vi "Breath.vi"() -> ()   [LabVIEW 2022 SP3]
uses:
  <vilib>/Analysis/NI_AALPro.lvlib
  <vilib>/Analysis/2dsp.llb/1D Cross Correlation (DBL).vi
  <vilib>/Analysis/NI_AALBase.lvlib
  <vilib>/Analysis/baseanly.llb/Mean (DBL).vi
panel:
  in  "ExitSendCmd 2":bool
  in  "Folder to place data":path
  in  "Extra Pts for Corr":i32=250
  out "ROI Coords":T1
  in  "ExitSendCmd":bool
  out "Focus RF Pt":dbl
  out "Correlations for window":dbl[][](graph)
  out "Total RF shift for groups of 5":dbl[](graph)
  in  "ROC (mm)":i32=12
  out "Ref Image":dbl[][](graph)
  in  "Folder of data":path
  in  "pattern":string="*.eye"
  # "Only use with single sets of 25 in a folder for now."
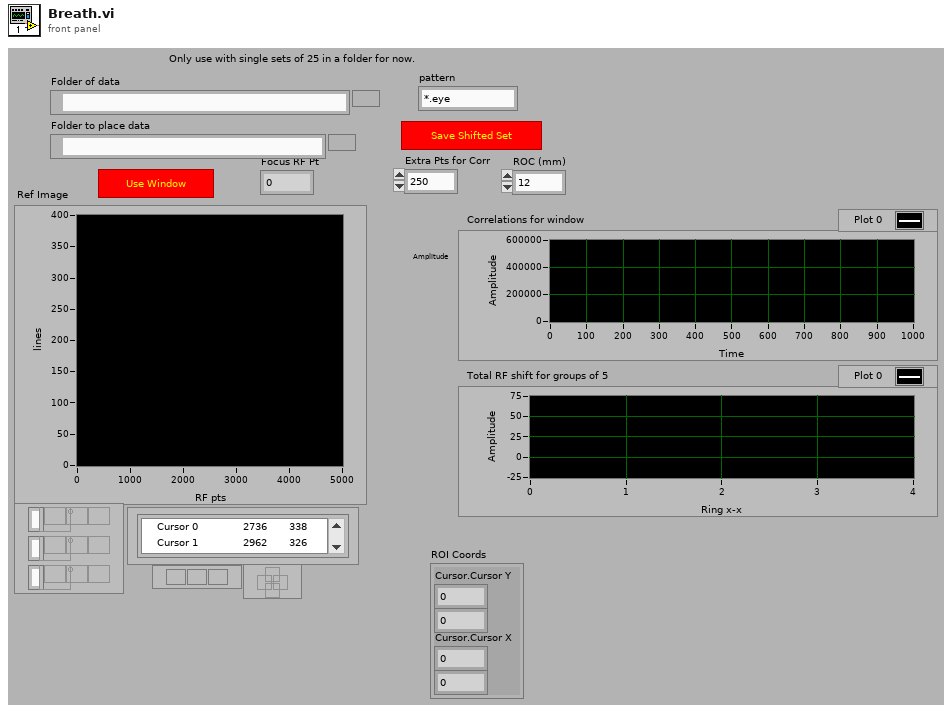
[diagram p1: front panel]
types:
  T1 = cluster{"Cursor.Cursor Y":dbl, dbl, "Cursor.Cursor X":dbl, dbl}
  T2 = cluster{"# rf points per line":u16, "# lines per scan":u16, "sample rate MHz":u16, "# A/D bits":u16, "# bytes per A/D":u16, "TGC Flag":u16, "A/D Type":string}
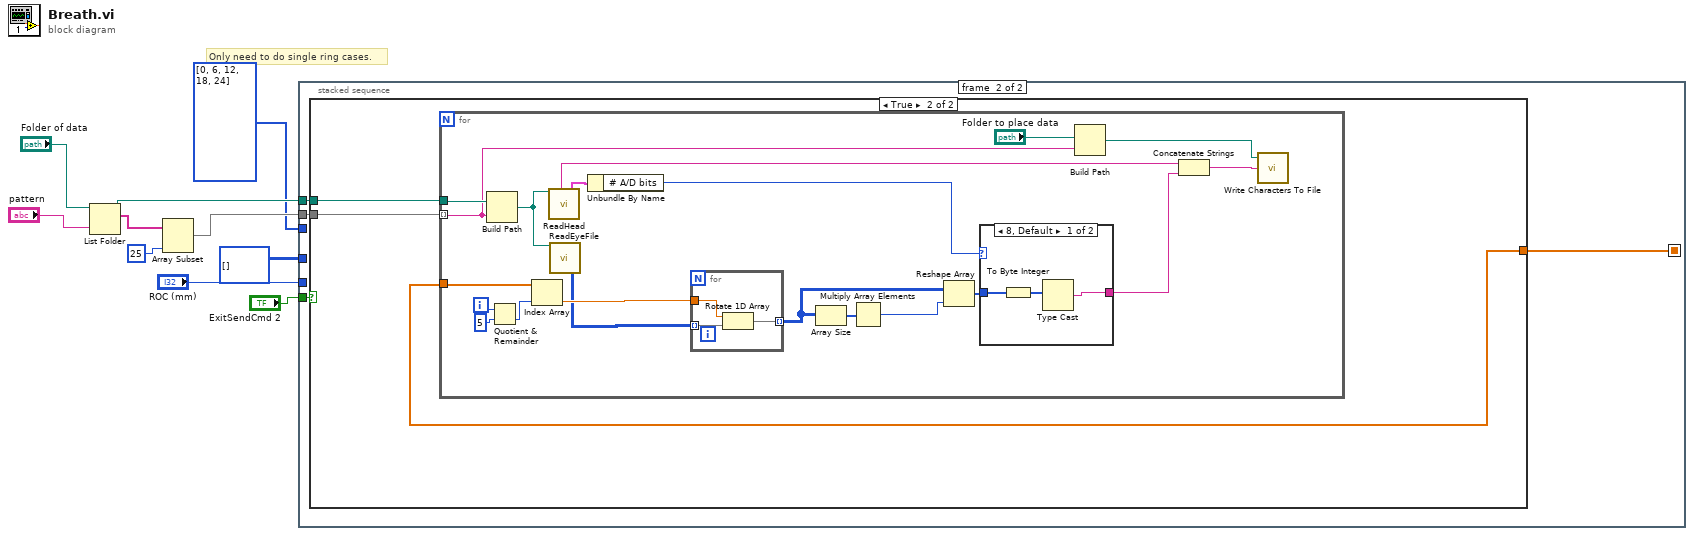
[diagram p0: block diagram]
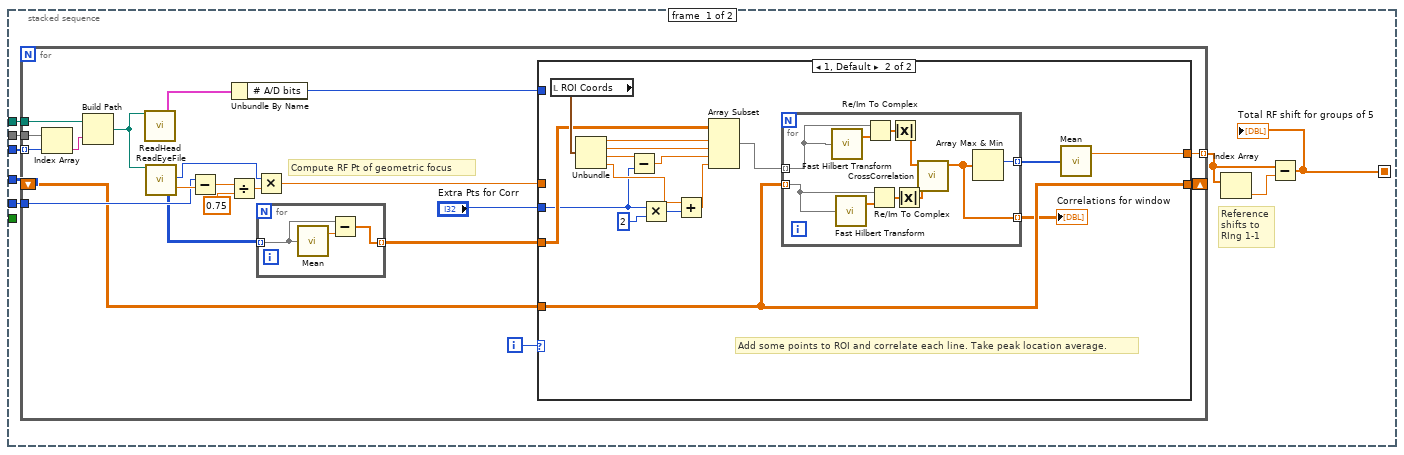
[diagram p2: hidden frame]
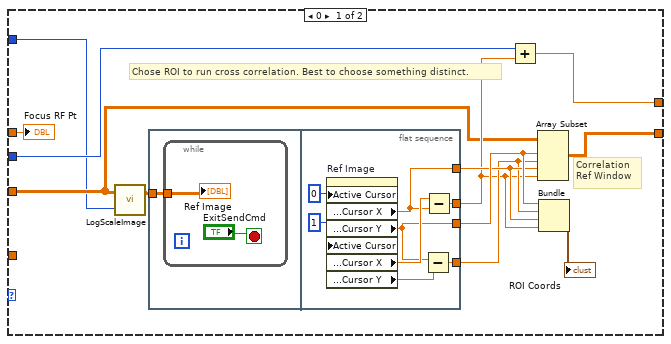
[diagram p3: hidden frame]
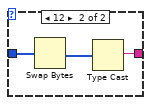
[diagram p5: hidden frame]
diagram:
  # "Only need to do single ring cases."
  n1 = List Folder(path="Folder of data", pattern="pattern") -> (path out=w8:path, filenames=w6:string[])  [unwired: 1 in, 3 out]
  n2 = Array Subset(array=w6, length=25) -> (w3:string[])  [unwired: 1 in]
  n3 = stacked-sequence {
    seq-local: [w11 _] -> [_ w93]
    tunnel: w8 -> [w18 w94]
    tunnel: "ROC (mm)" -> [w17 _]
    tunnel: i16[][] [] -> [w16 _]
    tunnel: w3 -> [w15 w95]
    tunnel: i32[] [0, 6, 12, 18, 24] -> [w14 _]
    tunnel: "ExitSendCmd 2" -> [_ w92]
    frame #0 {
      # "Reference shifts to RIng 1-1"
      n4 = for {
        tunnel: w15 -> [w22]
        tunnel: w18 -> [w39]
        tunnel: w17 -> [w35]
        shift-right: [w29] -> _
        shift-left: w16 -> [w28]
        tunnel: [w27] -> w12 mode=indexing
        tunnel: w14 -> [w20] mode=indexing
        i -> [w30]
        # "Compute RF Pt of geometric focus"
        n5 = Index Array(array=w22, index=w20) -> (element=w21:string)
        n6 = Build Path(base path=w39, name or relative path=w21) -> (appended path=w37:path)
        n7 = call "ReadHead.vi"("new file path"=w37) -> ("A/D info"=w38:T2)  [unwired: 18 out]
        n8 = call "ReadEyeFile.vi"("new file path"=w37) -> ("2-D data array"=w19:i16[][], "sample rate MHz"=w31:u16, "delay"=w36:sgl)  [unwired: 1 in, 15 out]
        n9 = Subtract(x=w35, y=w36) -> (x-y=w34:sgl)
        n10 = Divide(x=w34, y=0.75) -> (x/y=w32:dbl)
        n11 = Unbundle By Name(w38) -> ("# A/D bits"=w24:u16)
        n12 = Multiply(x=w31, y=w32) -> (x*y=w26:dbl)
        n13 = for {
          tunnel: [w41] -> w23 mode=indexing
          tunnel: w19 -> [w40] mode=indexing
          n14 = call-poly <vilib>:"Mean.vi"("X"=w40) -> ("mean"=w42:dbl)  [unwired: 1 out]
          n15 = Subtract(x=w40, y=w42) -> (x-y=w41:dbl[])
        }
        n16 = case shown="1, Default" w30 {
          tunnel: [w53 w81] -> w29
          tunnel: w28 -> [_ w81]
          tunnel: [w47 w80] -> w27
          tunnel: w26 -> [w54 _]
          tunnel: w23 -> [w45 w69]
          tunnel: "Extra Pts for Corr" -> [w49 w67]
          tunnel: w24 -> [w43 _]
          frame 0 {
            # "Correlation\nRef Window"
            # "Chose ROI to run cross correlation. Best to choose something distinct."
            n17 = call "LogScaleImage.vi"("A/D bits"=w43, "input array"=w45) -> ("log scale image"=w44:dbl[][])  [unwired: 1 out]
            n18 = flat-sequence {
              tunnel: w44 -> [w55]
              tunnel: [w61] -> w48
              tunnel: [w60] -> w52
              tunnel: [w59] -> w46
              tunnel: [w58] -> w51
              frame #0 {
                n19 = while {
                  tunnel: w55 -> [w56]
                  stop <- "ExitSendCmd" stop-if-true
                  "Ref Image" <- w56
                }
              }
              frame #1 {
                n20 = property on="Ref Image" class="IntGraph (strict)"("Active Cursor"=0, "Active Cursor"=1) -> ("Cursor.Cursor Position:Cursor X"=w58:dbl, "Cursor.Cursor Position:Cursor Y"=w60:dbl, "Cursor.Cursor Position:Cursor X"=w63:dbl, "Cursor.Cursor Position:Cursor Y"=w62:dbl)  [unwired: 2 in, 2 out]
                n21 = Subtract(x=w60, y=w62) -> (x-y=w61:dbl)
                n22 = Subtract(x=w63, y=w58) -> (x-y=w59:dbl)
              }
            }
            n23 = Add(x=w49, y=w46) -> (x+y=w47:dbl)
            n24 = Array Subset(array=w45, index (row)=w52, length (row)=w48, index (col)=w51, length (col)=w46) -> (w53:dbl[][])
            n25 = Bundle("Cursor.Cursor Y"=w52, w48, "Cursor.Cursor X"=w51, w46) -> (→"ROI Coords":T1)  [unwired: 1 out]
            "Focus RF Pt" <- w54
          }
          frame 1, Default {
            # "Add some points to ROI and correlate each line. Take peak location average."
            n26 = local read "ROI Coords"() -> (w78:T1)
            n27 = Unbundle(w78) -> ("Cursor.Cursor Y"=w77:dbl, w76:dbl, "Cursor.Cursor X"=w75:dbl, w71:dbl)
            n28 = Subtract(x=w75, y=w67) -> (x-y=w74:dbl)
            n29 = Multiply(x=w67, y=2) -> (x*y=w72:i32)
            n30 = Add(x=w71, y=w72) -> (x+y=w70:dbl)
            n31 = Array Subset(array=w69, index (row)=w77, length (row)=w76, index (col)=w74, length (col)=w70) -> (w68:dbl[][])
            n32 = for {
              tunnel: w68 -> [w84] mode=indexing
              tunnel: w81 -> [w85] mode=indexing
              tunnel: [w91] -> w79 mode=indexing
              tunnel: [w90] -> w66 mode=indexing
              n33 = call <vilib>:"Fast Hilbert Transform.vi"("X"=w84) -> ("Hilbert{X}"=w89:dbl[])  [unwired: 1 out]
              n34 = call <vilib>:"Fast Hilbert Transform.vi"("X"=w85) -> ("Hilbert{X}"=w87:dbl[])  [unwired: 1 out]
              n35 = Re/Im To Complex(1:w89, 2:w84) -> (0:w88:cdb[])
              n36 = Re/Im To Complex(1:w87, 2:w85) -> (0:w86:cdb[])
              n37 = Absolute Value(x=w88) -> (abs(x)=w83:dbl[])
              n38 = Absolute Value(x=w86) -> (abs(x)=w82:dbl[])
              n39 = call-poly <vilib>:"CrossCorrelation.vi"("Y"=w82, "X"=w83) -> ("Rxy"=w90:dbl[])  [unwired: 2 in, 7 out]
              n40 = Array Max & Min(array=w90) -> (max index (indices)=w91:i32)  [unwired: 3 out]
            }
            "Correlations for window" <- w66
            n41 = call-poly <vilib>:"Mean.vi"("X"=w79) -> ("mean"=w80:dbl)  [unwired: 1 out]
          }
        }
      }
      n42 = Index Array(array=w12) -> (element=w13:dbl)  [unwired: 1 in]
      n43 = Subtract(x=w12, y=w13) -> (x-y=w11:dbl[])
      "Total RF shift for groups of 5" <- w11
    }
    frame #1 {
      n44 = case shown="True" w92 {
        tunnel: w95 -> [_ w98]
        tunnel: w94 -> [_ w97]
        tunnel: w93 -> [_ w96]
        frame False {
        }
        frame True {
          n45 = for {
            tunnel: w98 -> [w102] mode=indexing
            tunnel: w97 -> [w117]
            tunnel: w96 -> [w108]
            i -> [w109]
            n46 = Build Path(base path=w117, name or relative path=w102) -> (appended path=w118:path)
            n47 = Quotient & Remainder(x=w109, y=5) -> (floor(x/y)=w107:i32)  [unwired: 1 out]
            n48 = Index Array(array=w108, index=w107) -> (element=w106:dbl)
            n49 = call "ReadHead.vi"("new file path"=w118) -> ("whole header"=w105:string, "A/D info"=w112:T2)  [unwired: 17 out]
            n50 = call "ReadEyeFile.vi"("new file path"=w118) -> ("2-D data array"=w99:i16[][])  [unwired: 1 in, 17 out]
            n51 = Unbundle By Name(w112) -> ("# A/D bits"=w111:u16)
            n52 = for {
              tunnel: w99 -> [w127] mode=indexing
              tunnel: [w126] -> w113 mode=indexing
              tunnel: w106 -> [w125]
              n53 = Rotate 1D Array(1:w127, 2:w125) -> (0:w126:i16[])
            }
            n54 = Array Size(array=w113) -> (size(s)=w115:i32[])
            n55 = Multiply Array Elements(1:w115) -> (0:w104:i32)
            n56 = Reshape Array(w113, w104) -> (w116:i16[])
            n57 = case shown="8, Default" w111 {
              tunnel: w116 -> [w120 w124]
              tunnel: [w121 w123] -> w114
              frame 8, Default {
                n58 = To Byte Integer(number=w120) -> (8bit integer=w119:i8[])
                n59 = Type Cast(x=w119) -> (*(type *) &x=w121:string)  [unwired: 1 out]
              }
              frame 12 {
                n60 = Swap Bytes(anything=w124) -> (byte swapped=w122:i16[])
                n61 = Type Cast(x=w122) -> (*(type *) &x=w123:string)  [unwired: 1 out]
              }
            }
            n62 = Build Path(base path="Folder to place data", name or relative path=w102) -> (appended path=w101:path)
            n63 = Concatenate Strings(w105, w114) -> (w103:string)
            n64 = call <vilib>:"Write Characters To File.vi"("character string"=w103, "file path (dialog if empty)"=w101) -> ()  [unwired: 1 in, 3 out]
          }
        }
      }
    }
  }
